vi "getVIRef.vi"(8 "error in (no error)":errorcluster, 11 "TaskName":string) -> (0 "error out":errorcluster, 2 "Task Ref":refnum<vi>, 3 "TaskName out":string)   [LabVIEW 2015, in "pdbm_task_route.lvlib"]
uses:
  pdbm_task_route.lvlib
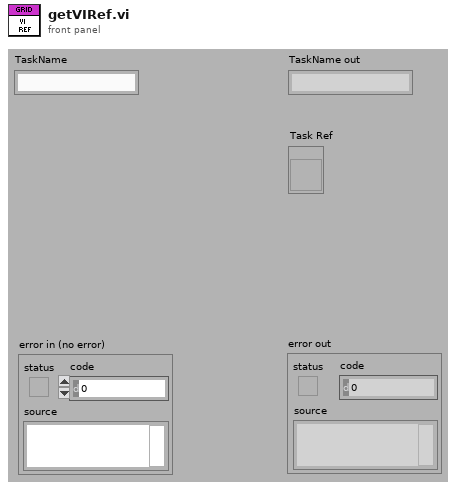
[diagram p1: front panel]
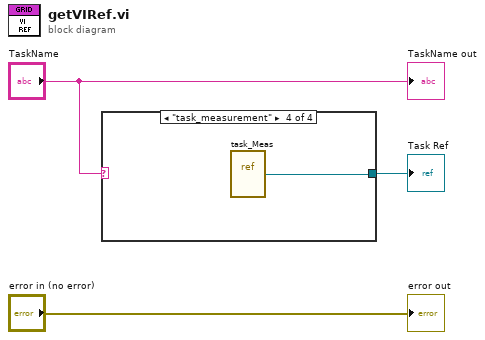
[diagram p0: block diagram]
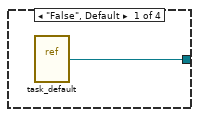
[diagram p2: hidden frame]
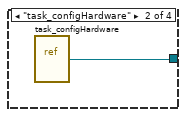
[diagram p3: hidden frame]
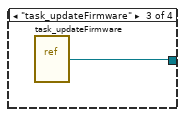
[diagram p4: hidden frame]
diagram:
  n1 = case shown="\"task_measurement\"" "TaskName" {
    tunnel: [w4 w5 w6 w7] -> w1
    frame "False", Default {
      n2 = vi-ref "task_default.vi"() -> (w4:refnum<vi>)
    }
    frame "task_configHardware" {
      n3 = vi-ref "task_configHardware.vi"() -> (w5:refnum<vi>)
    }
    frame "task_updateFirmware" {
      n4 = vi-ref "task_updateFirmware.vi"() -> (w6:refnum<vi>)
    }
    frame "task_measurement" {
      n5 = vi-ref "task_Meas.vi"() -> (w7:refnum<vi>)
    }
  }
  "Task Ref" <- w1
  "error out" <- "error in (no error)"
  "TaskName out" <- "TaskName"
